vi "Triangle Search.vi"(0 "X":dbl[](array[numeric]), 5 "Y":dbl[](array[numeric]), 7 "Triangles":i32[][](array[numeric]), 9 "Xi":dbl[](array[numeric]), 11 "Yi":dbl[](array[numeric])) -> (8 "indices":dbl[](array[numeric]), 15 "error":i32)   [LabVIEW 2020, in "NI_AAL_Geometry.lvlib"]
uses:
  <vilib>/Analysis/NI_AAL_Geometry.lvlib
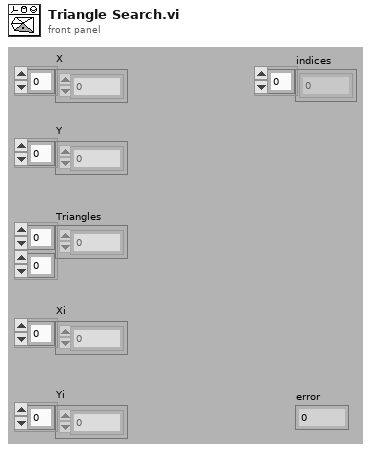
[diagram p1: front panel]
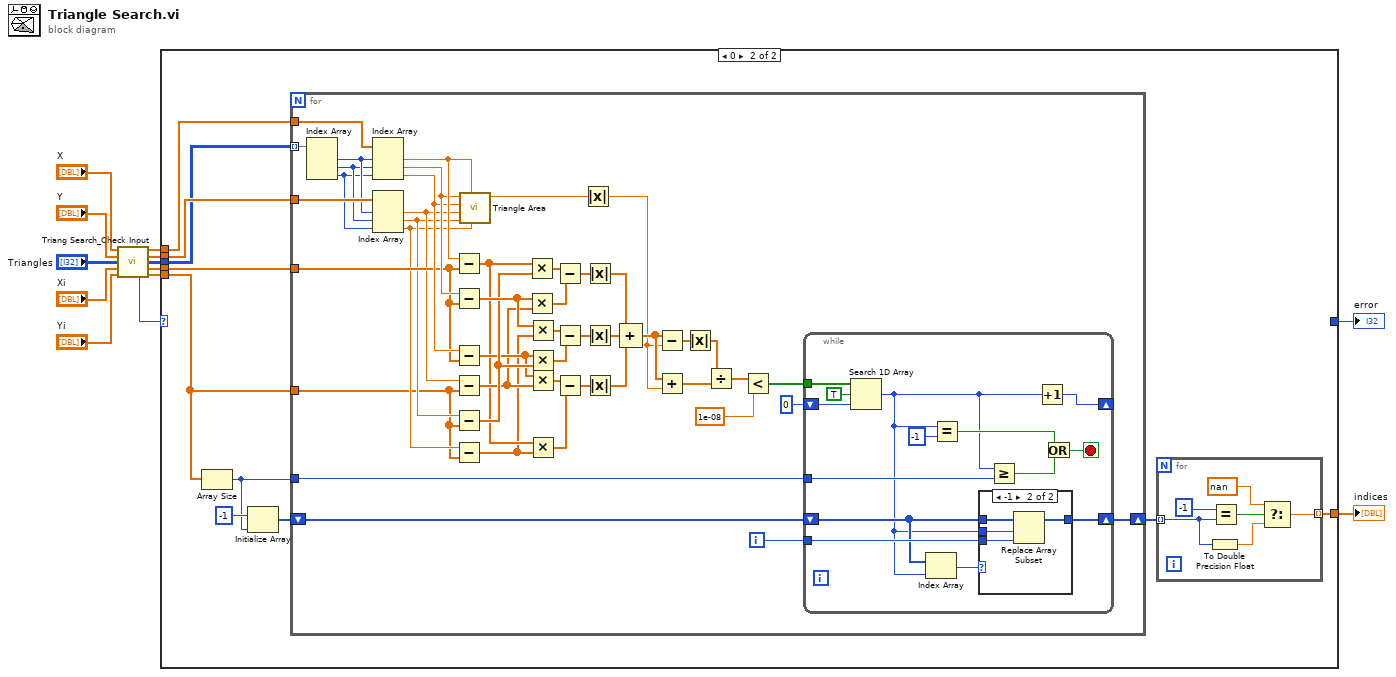
[diagram p0: block diagram]
diagram:
  n1 = call <vilib>:"Triang Search_Check Input.vi"("X In"="X", "Y In"="Y", "Triangles In"="Triangles", "Xi"="Xi", "Yi"="Yi") -> ("X Out"=w8:dbl[], "Y Out"=w7:dbl[], "Triangles Out"=w6:i32[][], "Xi Out"=w5:dbl[], "error"=w3:i32, "Yi Out"=w4:dbl[])  [unwired: 5 out]
  n2 = case shown="0" w3 {
    selector: w3 -> [w14 _]
    tunnel: [_ w16] -> w1
    tunnel: w8 -> [_ w22]
    tunnel: w7 -> [_ w23]
    tunnel: w6 -> [_ w21]
    tunnel: w5 -> [_ w24]
    tunnel: w4 -> [_ w20]
    tunnel: [w14 _] -> w2
    frame -1, Default {
    }
    frame 0 {
      n3 = Array Size(array=w20) -> (size(s)=w17:i32)
      n4 = Initialize Array(-1, w17) -> (w18:i32[])
      n5 = for {
        tunnel: w21 -> [w70] mode=indexing
        tunnel: w23 -> [w68]
        tunnel: w22 -> [w69]
        tunnel: w24 -> [w61]
        tunnel: w20 -> [w57]
        shift-right: [w25] -> w15
        shift-left: w18 -> [w27]
        tunnel: w17 -> [w28]
        i -> [w26]
        n6 = Index Array(array=w70) -> (element #1=w67:i32, element #2=w66:i32, element #3=w65:i32)  [unwired: 3 in]
        n7 = Index Array(array=w69, index #1=w67, index #2=w66, index #3=w65) -> (element #1=w64:dbl, element #2=w63:dbl, element #3=w62:dbl)
        n8 = Index Array(array=w68, index #1=w67, index #2=w66, index #3=w65) -> (element #1=w60:dbl, element #2=w59:dbl, element #3=w58:dbl)
        n9 = Subtract(x=w64, y=w61) -> (x-y=w46:dbl[])
        n10 = Subtract(x=w63, y=w61) -> (x-y=w54:dbl[])
        n11 = Subtract(x=w62, y=w61) -> (x-y=w48:dbl[])
        n12 = Subtract(x=w60, y=w57) -> (x-y=w47:dbl[])
        n13 = Subtract(x=w59, y=w57) -> (x-y=w53:dbl[])
        n14 = Subtract(x=w58, y=w57) -> (x-y=w45:dbl[])
        n15 = call <vilib>:"Triangle Area.vi"("y 3"=w58, "x 1"=w64, "y 2"=w59, "y 1"=w60, "x 3"=w62, "x 2"=w63) -> ("area"=w41:dbl)  [unwired: 5 in]
        n16 = Multiply(x=w46, y=w53) -> (x*y=w56:dbl[])
        n17 = Multiply(x=w54, y=w47) -> (x*y=w55:dbl[])
        n18 = Multiply(x=w54, y=w45) -> (x*y=w52:dbl[])
        n19 = Multiply(x=w48, y=w53) -> (x*y=w51:dbl[])
        n20 = Multiply(x=w48, y=w47) -> (x*y=w49:dbl[])
        n21 = Multiply(x=w46, y=w45) -> (x*y=w50:dbl[])
        n22 = Subtract(x=w56, y=w55) -> (x-y=w44:dbl[])
        n23 = Subtract(x=w52, y=w51) -> (x-y=w43:dbl[])
        n24 = Subtract(x=w49, y=w50) -> (x-y=w42:dbl[])
        n25 = Absolute Value(x=w41) -> (abs(x)=w31:dbl)
        n26 = Absolute Value(x=w44) -> (abs(x)=w40:dbl[])
        n27 = Absolute Value(x=w43) -> (abs(x)=w39:dbl[])
        n28 = Absolute Value(x=w42) -> (abs(x)=w38:dbl[])
        n29 = Compound Arithmetic op=ADD(w40, w39, w38) -> (w32:dbl[])
        n30 = Subtract(x=w32, y=w31) -> (x-y=w37:dbl[])
        n31 = Add(x=w32, y=w31) -> (x+y=w35:dbl[])
        n32 = Absolute Value(x=w37) -> (abs(x)=w34:dbl[])
        n33 = Divide(x=w34, y=w35) -> (x/y=w33:dbl[])
        n34 = Less?(x=w33, y=1e-08) -> (x < y?=w30:bool[])
        n35 = while {
          tunnel: w30 -> [w84]
          shift-right: [w81] -> _
          shift-left: 0 -> [w82]
          tunnel: w28 -> [w79]
          shift-right: [w75] -> w25
          shift-left: w27 -> [w73]
          tunnel: w26 -> [w74]
          stop <- w76 stop-if-true
          n36 = Search 1D Array(1D array=w84, element=TRUE, start index (0)=w82) -> (index of element=w72:i32)
          n37 = Index Array(array=w73, index=w72) -> (element=w71:i32)
          n38 = Equal?(x=w72, y=-1) -> (x = y?=w77:bool)
          n39 = case shown="-1" w71 {
            tunnel: [w85 w89] -> w75
            tunnel: w74 -> [_ w88]
            tunnel: w73 -> [w85 w87]
            tunnel: w72 -> [_ w86]
            frame Default {
            }
            frame -1 {
              n40 = Replace Array Subset(array=w87, new element=w88, index=w86) -> (w89:i32[])
            }
          }
          n41 = Greater Or Equal?(x=w72, y=w79) -> (x >= y?=w78:bool)
          n42 = Increment(x=w72) -> (x+1=w81:i32)
          n43 = Or(x=w77, y=w78) -> (x .or. y?=w76:bool)
        }
      }
      n44 = for {
        tunnel: w15 -> [w90] mode=indexing
        tunnel: [w92] -> w16 mode=indexing
        n45 = To Double Precision Float(number=w90) -> (double precision float=w91:dbl)
        n46 = Equal?(x=-1 ("y"), y=w90) -> (x = y?=w94:bool)
        n47 = Select(t=nan, s=w94, f=w91) -> (s? t:f=w92:dbl)
      }
    }
  }
  "indices" <- w1
  "error" <- w2
